vi "DoCreateError.vi"(5 "MergeErrors":bool, 6 "AdditionalText":string, 7 "Data":variant, 8 "ErrorIn":errorcluster caption="Error In", 9 "Text":string, 10 "ErrorCode":i32, 11 "ObjectIn":refnum<class "ErrorCreationExecution.lvclass"> caption="Object In") -> (0 "ErrorOut":errorcluster caption="Error Out", 3 "ObjectOut":refnum<class "ErrorCreationExecution.lvclass"> caption="Object Out")   [LabVIEW 2021, in "ErrorCreationExecution.lvclass"]
uses:
  ErrorCreationExecution.lvclass
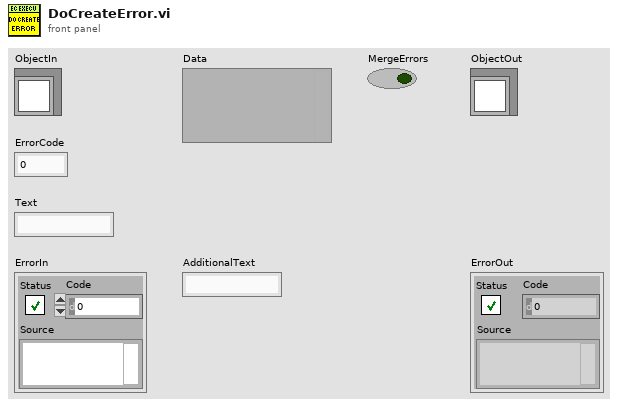
[diagram p1: front panel]
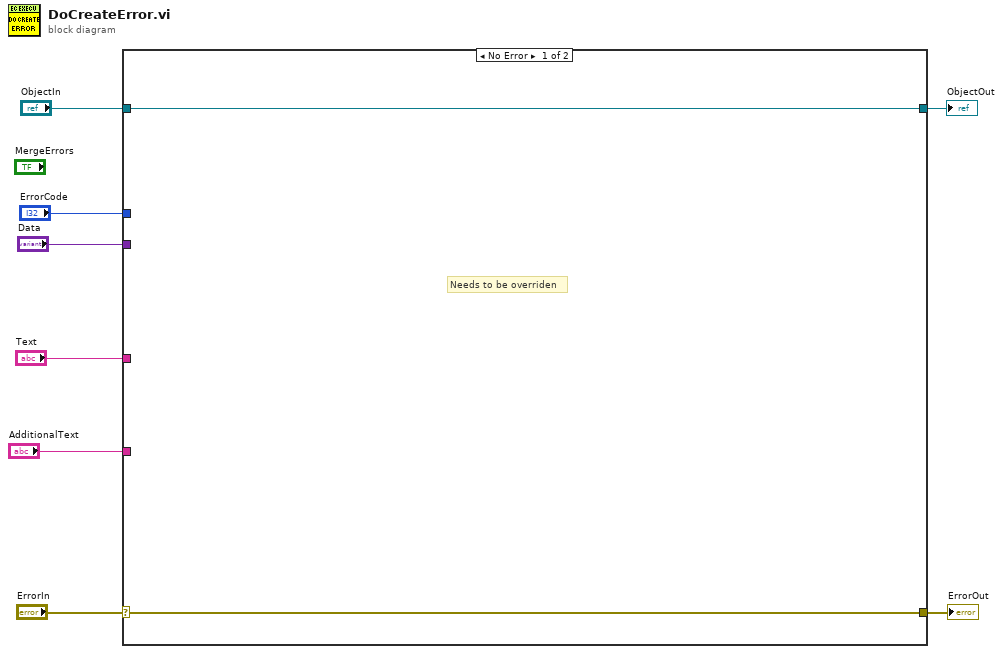
[diagram p0: block diagram]
diagram:
  n1 = case shown="No Error" "ErrorIn" {
    selector: "ErrorIn" -> [w9 w12]
    tunnel: [w9 w12] -> w7
    tunnel: [w10 w11] -> w5
    tunnel: "ObjectIn" -> [w10 w11]
    tunnel: "AdditionalText" -> [_ _]
    tunnel: "Text" -> [_ _]
    tunnel: "ErrorCode" -> [_ _]
    tunnel: "Data" -> [_ _]
    frame No Error {
      # "Needs to be overriden"
    }
    frame Error {
    }
  }
  "ErrorOut" <- w7
  "ObjectOut" <- w5
